vi "Engine-Event-KeyUp.vi"(6 "Key":T2 {"Mod" items=["SDL_KMOD_NONE"=0, "SDL_KMOD_LSHIFT"=1, "SDL_KMOD_RSHIFT"=2, "SDL_KMOD_LCTRL"=64, "SDL_KMOD_RCTRL"=128, "SDL_KMOD_LALT"=256, "SDL_KMOD_RALT"=512, "SDL_KMOD_LGUI"=1024, "SDL_KMOD_RGUI"=2048, "SDL_KMOD_NUM"=4096, "SDL_KMOD_CAPS"=8192, "SDL_KMOD_MODE"=16384, "SDL_KMOD_SCROLL"=32768, "SDL_KMOD_CTRL"=192, "SDL_KMOD_SHIFT"=3, "SDL_KMOD_ALT"=768, "SDL_KMOD_GUI"=3072]; "Keycode" items=["SDLK_SCANCODE_MASK"=1073741824, "SDLK_UNKNOWN"=0, "SDLK_RETURN"=13, "SDLK_ESCAPE"=27, "SDLK_BACKSPACE"=8, "SDLK_TAB"=9, "SDLK_SPACE"=32, "SDLK_EXCLAIM"=33, "SDLK_DBLAPOSTROPHE"=34, "SDLK_HASH"=35, "SDLK_DOLLAR"=36, "SDLK_PERCENT"=37, "SDLK_AMPERSAND"=38, "SDLK_APOSTROPHE"=39, "SDLK_LEFTPAREN"=40, "SDLK_RIGHTPAREN"=41, "SDLK_ASTERISK"=42, "SDLK_PLUS"=43, "SDLK_COMMA"=44, "SDLK_MINUS"=45, "SDLK_PERIOD"=46, "SDLK_SLASH"=47, "SDLK_0"=48, "SDLK_1"=49, "SDLK_2"=50, "SDLK_3"=51, "SDLK_4"=52, "SDLK_5"=53, "SDLK_6"=54, "SDLK_7"=55, "SDLK_8"=56, "SDLK_9"=57, "SDLK_COLON"=58, "SDLK_SEMICOLON"=59, "SDLK_LESS"=60, "SDLK_EQUALS"=61, "SDLK_GREATER"=62, "SDLK_QUESTION"=63, "SDLK_AT"=64, "SDLK_LEFTBRACKET"=91, "SDLK_BACKSLASH"=92, "SDLK_RIGHTBRACKET"=93, "SDLK_CARET"=94, "SDLK_UNDERSCORE"=95, "SDLK_GRAVE"=96, "SDLK_A"=97, "SDLK_B"=98, "SDLK_C"=99, "SDLK_D"=100, "SDLK_E"=101, "SDLK_F"=102, "SDLK_G"=103, "SDLK_H"=104, "SDLK_I"=105, "SDLK_J"=106, "SDLK_K"=107, "SDLK_L"=108, "SDLK_M"=109, "SDLK_N"=110, "SDLK_O"=111, "SDLK_P"=112, "SDLK_Q"=113, "SDLK_R"=114, "SDLK_S"=115, "SDLK_T"=116, "SDLK_U"=117, "SDLK_V"=118, "SDLK_W"=119, "SDLK_X"=120, "SDLK_Y"=121, "SDLK_Z"=122, "SDLK_LEFTBRACE"=123, "SDLK_PIPE"=124, "SDLK_RIGHTBRACE"=125, "SDLK_TILDE"=126, "SDLK_DELETE"=127, "SDLK_PLUSMINUS"=177, "SDLK_CAPSLOCK"=1073741881, "SDLK_F1"=1073741882, "SDLK_F2"=1073741883, "SDLK_F3"=1073741884, "SDLK_F4"=1073741885, "SDLK_F5"=1073741886, "SDLK_F6"=1073741887, "SDLK_F7"=1073741888, "SDLK_F8"=1073741889, "SDLK_F9"=1073741890, "SDLK_F10"=1073741891, "SDLK_F11"=1073741892, "SDLK_F12"=1073741893, "SDLK_PRINTSCREEN"=1073741894, "SDLK_SCROLLLOCK"=1073741895, "SDLK_PAUSE"=1073741896, "SDLK_INSERT"=1073741897, "SDLK_HOME"=1073741898, "SDLK_PAGEUP"=1073741899, "SDLK_END"=1073741901, "SDLK_PAGEDOWN"=1073741902, "SDLK_RIGHT"=1073741903, "SDLK_LEFT"=1073741904, "SDLK_DOWN"=1073741905, "SDLK_UP"=1073741906, "SDLK_NUMLOCKCLEAR"=1073741907, "SDLK_KP_DIVIDE"=1073741908, "SDLK_KP_MULTIPLY"=1073741909, "SDLK_KP_MINUS"=1073741910, "SDLK_KP_PLUS"=1073741911, "SDLK_KP_ENTER"=1073741912, "SDLK_KP_1"=1073741913, "SDLK_KP_2"=1073741914, "SDLK_KP_3"=1073741915, "SDLK_KP_4"=1073741916, "SDLK_KP_5"=1073741917, "SDLK_KP_6"=1073741918, "SDLK_KP_7"=1073741919, "SDLK_KP_8"=1073741920, "SDLK_KP_9"=1073741921, "SDLK_KP_0"=1073741922, "SDLK_KP_PERIOD"=1073741923, "SDLK_APPLICATION"=1073741925, "SDLK_POWER"=1073741926, "SDLK_KP_EQUALS"=1073741927, "SDLK_F13"=1073741928, "SDLK_F14"=1073741929, "SDLK_F15"=1073741930, "SDLK_F16"=1073741931, "SDLK_F17"=1073741932, "SDLK_F18"=1073741933, "SDLK_F19"=1073741934, "SDLK_F20"=1073741935, "SDLK_F21"=1073741936, "SDLK_F22"=1073741937, "SDLK_F23"=1073741938, "SDLK_F24"=1073741939, "SDLK_EXECUTE"=1073741940, "SDLK_HELP"=1073741941, "SDLK_MENU"=1073741942, "SDLK_SELECT"=1073741943, "SDLK_STOP"=1073741944, "SDLK_AGAIN"=1073741945, "SDLK_UNDO"=1073741946, "SDLK_CUT"=1073741947, "SDLK_COPY"=1073741948, "SDLK_PASTE"=1073741949, "SDLK_FIND"=1073741950, "SDLK_MUTE"=1073741951, "SDLK_VOLUMEUP"=1073741952, "SDLK_VOLUMEDOWN"=1073741953, "SDLK_KP_COMMA"=1073741957, "SDLK_KP_EQUALSAS400"=1073741958, "SDLK_ALTERASE"=1073741977, "SDLK_SYSREQ"=1073741978, "SDLK_CANCEL"=1073741979, "SDLK_CLEAR"=1073741980, "SDLK_PRIOR"=1073741981, "SDLK_RETURN2"=1073741982, "SDLK_SEPARATOR"=1073741983, "SDLK_OUT"=1073741984, "SDLK_OPER"=1073741985, "SDLK_CLEARAGAIN"=1073741986, "SDLK_CRSEL"=1073741987, "SDLK_EXSEL"=1073741988, "SDLK_KP_00"=1073742000, "SDLK_KP_000"=1073742001, "SDLK_THOUSANDSSEPARATOR"=1073742002, "SDLK_DECIMALSEPARATOR"=1073742003, "SDLK_CURRENCYUNIT"=1073742004, "SDLK_CURRENCYSUBUNIT"=1073742005, "SDLK_KP_LEFTPAREN"=1073742006, "SDLK_KP_RIGHTPAREN"=1073742007, "SDLK_KP_LEFTBRACE"=1073742008, "SDLK_KP_RIGHTBRACE"=1073742009, "SDLK_KP_TAB"=1073742010, "SDLK_KP_BACKSPACE"=1073742011, "SDLK_KP_A"=1073742012, "SDLK_KP_B"=1073742013, "SDLK_KP_C"=1073742014, "SDLK_KP_D"=1073742015, "SDLK_KP_E"=1073742016, "SDLK_KP_F"=1073742017, "SDLK_KP_XOR"=1073742018, "SDLK_KP_POWER"=1073742019, "SDLK_KP_PERCENT"=1073742020, "SDLK_KP_LESS"=1073742021, "SDLK_KP_GREATER"=1073742022, "SDLK_KP_AMPERSAND"=1073742023, "SDLK_KP_DBLAMPERSAND"=1073742024, "SDLK_KP_VERTICALBAR"=1073742025, "SDLK_KP_DBLVERTICALBAR"=1073742026, "SDLK_KP_COLON"=1073742027, "SDLK_KP_HASH"=1073742028, "SDLK_KP_SPACE"=1073742029, "SDLK_KP_AT"=1073742030, "SDLK_KP_EXCLAM"=1073742031, "SDLK_KP_MEMSTORE"=1073742032, "SDLK_KP_MEMRECALL"=1073742033, "SDLK_KP_MEMCLEAR"=1073742034, "SDLK_KP_MEMADD"=1073742035, "SDLK_KP_MEMSUBTRACT"=1073742036, "SDLK_KP_MEMMULTIPLY"=1073742037, "SDLK_KP_MEMDIVIDE"=1073742038, "SDLK_KP_PLUSMINUS"=1073742039, "SDLK_KP_CLEAR"=1073742040, "SDLK_KP_CLEARENTRY"=1073742041, "SDLK_KP_BINARY"=1073742042, "SDLK_KP_OCTAL"=1073742043, "SDLK_KP_DECIMAL"=1073742044, "SDLK_KP_HEXADECIMAL"=1073742045, "SDLK_LCTRL"=1073742048, "SDLK_LSHIFT"=1073742049, "SDLK_LALT"=1073742050, "SDLK_LGUI"=1073742051, "SDLK_RCTRL"=1073742052, "SDLK_RSHIFT"=1073742053, "SDLK_RALT"=1073742054, "SDLK_RGUI"=1073742055, "SDLK_MODE"=1073742081, "SDLK_SLEEP"=1073742082, "SDLK_WAKE"=1073742083, "SDLK_CHANNEL_INCREMENT"=1073742084, "SDLK_CHANNEL_DECREMENT"=1073742085, "SDLK_MEDIA_PLAY"=1073742086, "SDLK_MEDIA_PAUSE"=1073742087, "SDLK_MEDIA_RECORD"=1073742088, "SDLK_MEDIA_FAST_FORWARD"=1073742089, "SDLK_MEDIA_REWIND"=1073742090, "SDLK_MEDIA_NEXT_TRACK"=1073742091, "SDLK_MEDIA_PREVIOUS_TRACK"=1073742092, "SDLK_MEDIA_STOP"=1073742093, "SDLK_MEDIA_EJECT"=1073742094, "SDLK_MEDIA_PLAY_PAUSE"=1073742095, "SDLK_MEDIA_SELECT"=1073742096, "SDLK_AC_NEW"=1073742097, "SDLK_AC_OPEN"=1073742098, "SDLK_AC_CLOSE"=1073742099, "SDLK_AC_EXIT"=1073742100, "SDLK_AC_SAVE"=1073742101, "SDLK_AC_PRINT"=1073742102, "SDLK_AC_PROPERTIES"=1073742103, "SDLK_AC_SEARCH"=1073742104, "SDLK_AC_HOME"=1073742105, "SDLK_AC_BACK"=1073742106, "SDLK_AC_FORWARD"=1073742107, "SDLK_AC_STOP"=1073742108, "SDLK_AC_REFRESH"=1073742109, "SDLK_AC_BOOKMARKS"=1073742110, "SDLK_SOFTLEFT"=1073742111, "SDLK_SOFTRIGHT"=1073742112, "SDLK_CALL"=1073742113, "SDLK_ENDCALL"=1073742114]}, 8 "error in (no error)":errorcluster, 9 "Which":T1, 10 "Timestamp":u64, 11 "GLF Window in":refnum<class "Window.lvclass">) -> (0 "error out":errorcluster, 3 "GLF Window out":refnum<class "Window.lvclass">)   [LabVIEW 2020, in "GLF.lvlib" / "Window.lvclass"]
uses:
  Window.lvclass
  Window.lvclass/Window.ctl
  WindowEventInterface/WindowEventInterface.lvclass
  <vilib>/Saukko/LV SDL3/Sources/SDL3/Events/Scancode--integer.ctl
  <vilib>/Saukko/LV SDL3/Sources/SDL3/Events/Events.lvlib
  <vilib>/Saukko/LV SDL3/Sources/SDL3/Keycode/Keycode--ring.ctl
  <vilib>/Saukko/LV SDL3/Sources/SDL3/Keycode/Keycode.lvlib
  <vilib>/Saukko/LV SDL3/Sources/SDL3/Keycode/Keymod--ring.ctl
  WindowEventInterface/Key--cluster.ctl
  <vilib>/Saukko/LV SDL3/Sources/SDL3/Keyboard/KeyboardID--integer.ctl
  <vilib>/Saukko/LV SDL3/Sources/SDL3/Keyboard/Keyboard.lvlib
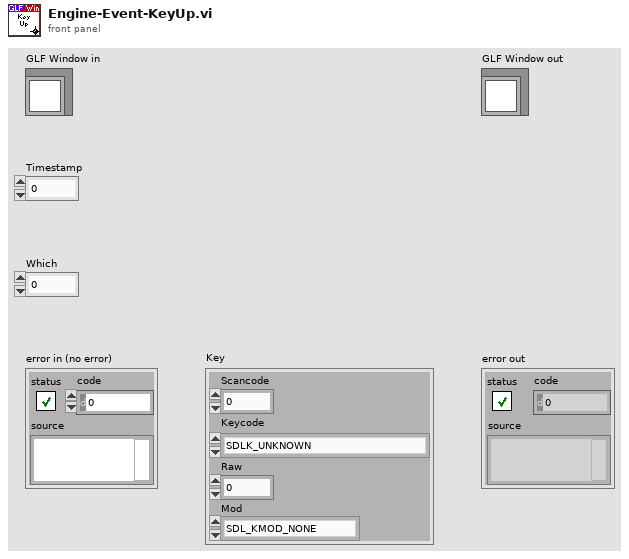
[diagram p1: front panel]
types:
  T1 = typedef "SDL3.lvlib/Keyboard.lvlib/KeyboardID--integer.ctl" = u32
  T2 = typedef "GLF.lvlib/WindowEventInterface.lvclass/Key--cluster.ctl" = cluster{"Scancode":T3, "Keycode":T4, "Raw":u16, "Mod":T5}
  T3 = typedef "SDL3.lvlib/Events.lvlib/Scancode--integer.ctl" = u32
  T4 = typedef "SDL3.lvlib/Keycode.lvlib/Keycode--ring.ctl" = u32
  T5 = typedef "SDL3.lvlib/Keycode.lvlib/Keymod--ring.ctl" = u16
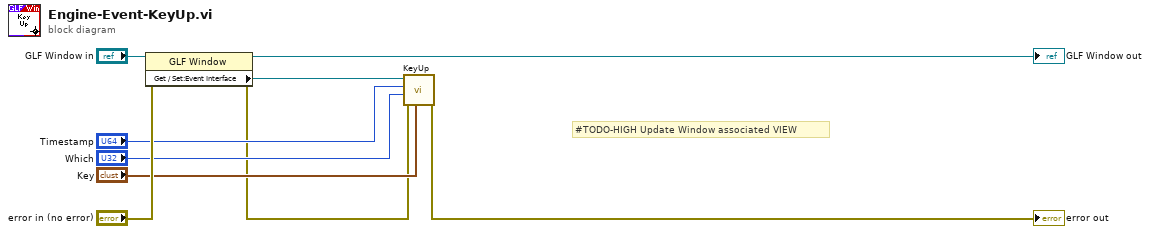
[diagram p0: block diagram]
diagram:
  # "#TODO-HIGH Update Window associated VIEW"
  n1 = property class="GLF Window"(reference="GLF Window in", error in="error in (no error)") -> (reference out=→"GLF Window out":refnum<class "Window.lvclass">, error out=w1:errorcluster, "Get / Set:Event Interface"=w6:refnum<class "WindowEventInterface.lvclass">)
  n2 = call-dynamic "KeyUp.vi"("Key"="Key", "error in (no error)"=w1, "Which"="Which", "Timestamp"="Timestamp", "WindowEventInterface in"=w6) -> ("error out"=→"error out":errorcluster)  [unwired: 6 in]
